vi "GetSoftwareVersion.vi"(8 "Fehler (Eingang, kein Fehler)":errorcluster caption="Error_In", 11 "OXYGEN Ref In":refnum<visa-resource-name>) -> (0 "Fehler (Ausgang)":errorcluster caption="Error_Out", 1 "Raw communication data":T1, 2 "Software Version Info":string, 3 "OXYGEN Ref Out":refnum<visa-resource-name>)   [LabVIEW 2018, in "OXYGEN.lvlib"]
doc: "Query the software and SCPI interface version string."
uses:
  OXYGEN.lvlib
  TypeDefs/Cluster_RawCommData.ctl
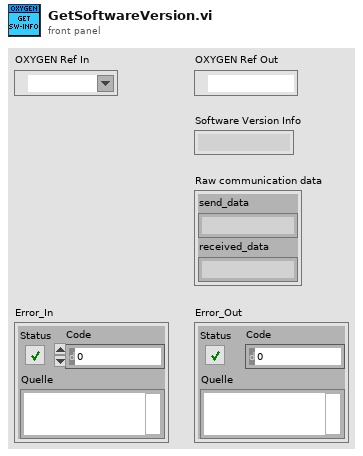
[diagram p1: front panel]
types:
  T1 = typedef "OXYGEN.lvlib/Cluster_RawCommData.ctl" = cluster{"send_data":string, "received_data":string}
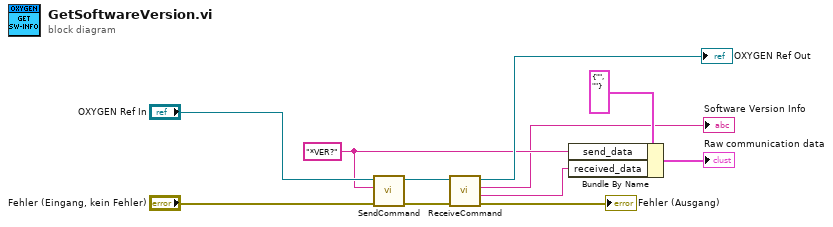
[diagram p0: block diagram]
diagram:
  w3 = "*VER?" ("Schreibpuffer")
  n1 = call "SendCommand.vi"("error in (no error)"="Fehler (Eingang, kein Fehler)", "String to Send"=w3, "OXY_SCPI Reseource In"="OXYGEN Ref In") -> ("error out"=w7:errorcluster, "OXY_SCPI Reseource Out"=w6:refnum<visa-resource-name>)  [unwired: 7 in]
  n2 = call "ReceiveCommand.vi"("error in (no error)"=w7, "OXY_SCPI Reseource In"=w6) -> ("error out"=→"Fehler (Ausgang)":errorcluster, "received Data with Header"=w1:string, "received Data"=→"Software Version Info":string, "OXY_SCPI Reseource Out"=→"OXYGEN Ref Out":refnum<visa-resource-name>)  [unwired: 6 in]
  n3 = Bundle By Name(cluster=T1 {"send_data"="", "received_data"=""} ("communication_data"), "send_data"=w3, "received_data"=w1) -> (→"Raw communication data":T1)
